vi "Convert Meta Data Parameters to RT.vi"(8 "error in (no error)":errorcluster, 9 "Data Index":i32, 10 "Item Ref in":T1 format="%.0x", 11 "Lookup Table":variant) -> (0 "error out":errorcluster, 2 "Chan Refs":T1[](array[typedef]) format="%.0x", 3 "Lookup Table out":variant)   [LabVIEW 2018, in "Instrument Addon System Explorer.lvlib"]
uses:
  Instrument Addon System Explorer.lvlib
  Addon Shared/Instrument Addon Shared.lvlib
  Addon Shared/Types/FG Control.ctl
  Addon Shared/Types/Metadata Channel Type.ctl
  Addon Shared/Types/Protocol Data Type.ctl
  Addon Shared/Types/MetaData Parameters.ctl
  Addon Shared/Types/Meta Data RT Configuration Cluster.ctl
  Addon Shared/SubVIs/Constants.vi
  <vilib>/NI VeriStand/Custom Device API/Custom Device API.lvlib
  <vilib>/NI VeriStand/Custom Device API/Get Item Property (String).vi
  Addon Shared/Types/Type Cast Type.ctl
  Addon Shared/Types/Endian.ctl
  <vilib>/NI VeriStand/Custom Device API/Custom Device Item Ref.ctl
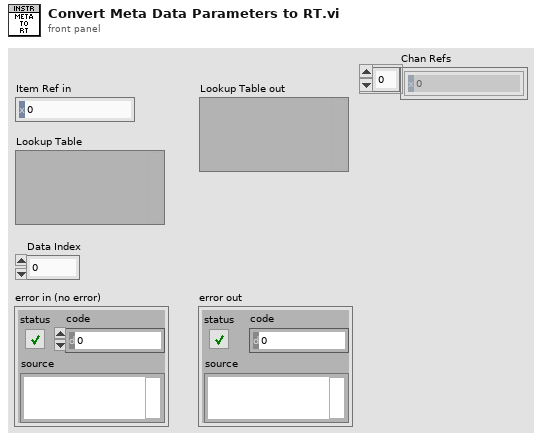
[diagram p1: front panel]
types:
  T1 = typedef "Custom Device API.lvlib/Custom Device Item Ref.ctl" = u64
  T2 = typedef "Instrument Addon Shared.lvlib/Meta Data RT Configuration Cluster.ctl" = cluster{"MetaData Parameters":T3, "Data Index":i32, "Data Length":i32}
  T3 = typedef "Instrument Addon Shared.lvlib/MetaData Parameters.ctl" = cluster{"Data Type":T4, "Channel Type":T5, "List":string[], "Format String":string, "Type":T6, "Delimiter":string, "Endian":T7}
  T4 = typedef "Instrument Addon Shared.lvlib/Protocol Data Type.ctl" = enum16{"Single Channel", "Array"}
  T5 = typedef "Instrument Addon Shared.lvlib/Metadata Channel Type.ctl" = enum16{"Enumerated List", "Format", "Type Cast"}
  T6 = typedef "Instrument Addon Shared.lvlib/Type Cast Type.ctl" = enum16{"DBL", "SGL", "U64", "U32", "U16", "U8", "I64", "I32", "I16", "I8"}
  T7 = typedef "Instrument Addon Shared.lvlib/Endian.ctl" = enum16{"Native", "Little", "Big"}
  T8 = typedef "Instrument Addon Shared.lvlib/FG Control.ctl" = enum16{"Get", "Set"}
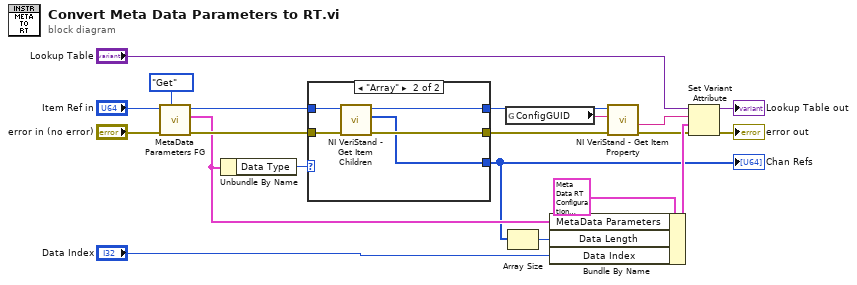
[diagram p0: block diagram]
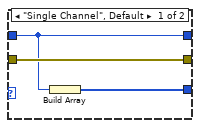
[diagram p2: hidden frame]
diagram:
  n1 = call "MetaData Parameters FG.vi"("Action"=FG_Control."Get", "error in (no error)"="error in (no error)", "Item Ref in"="Item Ref in") -> ("error out"=w7:errorcluster, "MetaData Parameters"=w5:T3, "Item Ref out"=w10:T1)  [unwired: 6 in]
  n2 = Unbundle By Name(w5) -> ("Data Type"=w4:T4)
  n3 = case shown="\"Array\"" w4 {
    tunnel: w10 -> [w22 w28]
    tunnel: [w22 w27] -> w8
    tunnel: w7 -> [w23 w26]
    tunnel: [w23 w25] -> w6
    tunnel: [w21 w24] -> w3
    frame "Single Channel", Default {
      n4 = Build Array(w22) -> (w21:T1[])
    }
    frame "Array" {
      n5 = call <vilib>:"NI VeriStand - Get Item Children.vi"("error in (no error)"=w26, "Item Ref in"=w28) -> ("error out"=w25:errorcluster, "Child Refs"=w24:T1[], "Item Ref out"=w27:T1)  [unwired: 6 in, 1 out]
    }
  }
  "Chan Refs" <- w3
  n6 = global read "Constants.vi" "ConfigGUID"() -> (w12:string)
  n7 = Array Size(array=w3) -> (size(s)=w2:i32)
  n8 = Bundle By Name(cluster=T2 {"MetaData Parameters"={"Data Type"=enum."Single Channel", "Channel Type"=enum."Enumerated List", "List"=[], "Format String"="", "Type"=enum."DBL", "Delimiter"="", "Endian"=enum."Native"}, "Data Index"=0, "Data Length"=0}, "MetaData Parameters"=w5, "Data Length"=w2, "Data Index"="Data Index") -> (w18:T2)
  n9 = call-poly <vilib>:"NI VeriStand - Get Item Property.vi"("error in (no error)"=w6, "Property Name"=w12, "Item Ref in"=w8) -> ("error out"=w11:errorcluster, "Value"=w9:string)  [unwired: 5 in, 2 out]
  n10 = Set Variant Attribute(Variant="Lookup Table", name=w9, value=w18, error in=w11) -> (Variant out=→"Lookup Table out":variant, error out=→"error out":errorcluster)  [unwired: 1 out]
